vi "c语言脚本以及cmd的python调用.vi"() -> ()   [LabVIEW 2020]
panel:
  in  "working directory":path=path "" caption="工作目录"
  out "standard error":string caption="标准错误"
  out "return code":i32 caption="返回代码"
  out "error out":errorcluster caption="错误输出"
  out "standard output":string caption="标准输出"
  out "输出变量":i32
  # "注意了嗷，需要自行配置python环境，或者使用绝对路径调用python.exe。懂得都懂"
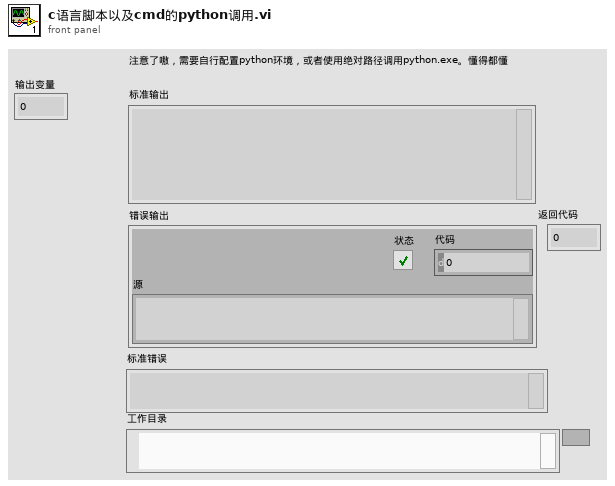
[diagram p1: front panel]
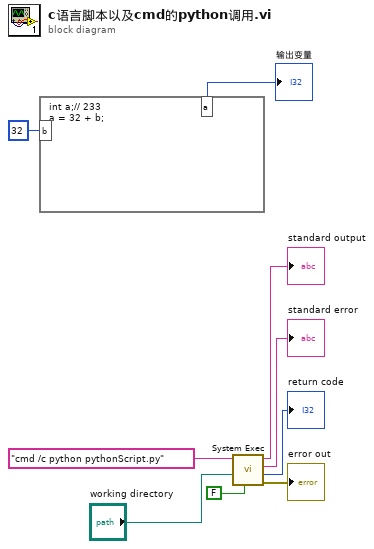
[diagram p0: block diagram]
diagram:
  n1 = formula code="int a;// 233\na = 32 + b;"("b"=32) -> ("a"=→"输出变量":i32)
  n2 = call <vilib>:"System Exec.vi"("run minimized? (F)"=FALSE, "working directory"="working directory", "command line"="cmd /c python pythonScript.py") -> ("error out"=→"error out":errorcluster, "return code"=→"return code":i32, "standard error"=→"standard error":string, "standard output"=→"standard output":string)  [unwired: 5 in]
